vi "GetParentInterfaces.vi"(0 "ClassReaderNative in":refnum<class "ClassReaderNative.lvclass">, 5 "error in (no error)":errorcluster) -> (14 "ClassReaderNative out":refnum<class "ClassReaderNative.lvclass">, 15 "ParentInterfaces":path[](array[path]), 19 "error out":errorcluster)   [LabVIEW 2020, in "ClassReaderNative.lvclass"]
uses:
  <resource>/Framework/Providers/Open_GDS/ClassProviders/Provider_LvNativeClass/ClassReaderNative_class/ClassReaderNative.lvclass
  <resource>/Framework/Providers/Open_GDS/ClassProviders/Provider_LvNativeClass/ClassReaderNative_class/ClassReaderNative.lvclass/ClassReaderNative.ctl
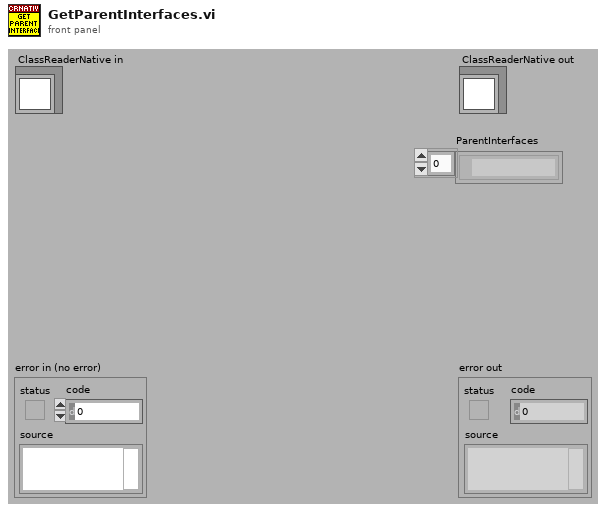
[diagram p1: front panel]
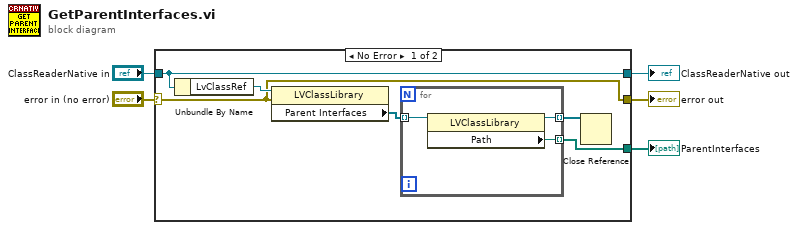
[diagram p0: block diagram]
diagram:
  n1 = case shown="No Error" "error in (no error)" {
    selector: "error in (no error)" -> [w6 w16]
    tunnel: [w11 _] -> w5
    tunnel: "ClassReaderNative in" -> [w7 w15]
    tunnel: [w6 w16] -> w2
    tunnel: [w7 w15] -> w1
    frame No Error {
      n2 = Unbundle By Name(w7) -> ("LvClassRef"=w9:refnum<vi>)
      n3 = property class="LVClassLibrary"(reference=w9, error in=w6) -> ("Parent Interfaces"=w10:refnum<vi>[])  [unwired: 2 out]
      n4 = for {
        tunnel: w10 -> [w14] mode=indexing
        tunnel: [w13] -> w11 mode=indexing
        tunnel: [w12] -> w8 mode=indexing
        n5 = property class="LVClassLibrary"(reference=w14) -> (reference out=w12:refnum<vi>, "Path"=w13:path)  [unwired: 1 in, 1 out]
      }
      n6 = Close Reference(reference=w8) -> ()  [unwired: 1 in, 1 out]
    }
    frame Error {
    }
  }
  "ClassReaderNative out" <- w1
  "ParentInterfaces" <- w5
  "error out" <- w2
